vi "apresentacao.vi"() -> ()   [LabVIEW 2016]
uses:
  <vilib>/NXT/Subs/LVHSConnector.ctl
  <vilib>/NXT/LegoClasses/BrickReference/BrickReference.lvclass
  <vilib>/NXT/Block Support/NXT_InputPort.ctl
  <vilib>/NXT/Block Support/NXT_ButtonSelector.ctl
  <vilib>/NXT/Block Support/NXT_OutputPort.ctl
  <vilib>/NXT/Dual Mode Library/Advanced/NXTFlag_Clear.vi
  <vilib>/NXT/Dual Mode Library/Advanced/NXTFlag_Get_String.vi
  <vilib>/NXT/Dual Mode Library/Display/drawText_Center.vi
  <vilib>/NXT/Dual Mode Library/Advanced/NXTFlag_Get.vi
  <vilib>/NXT/Dual Mode Library/Advanced/NXTFlag_Clear_String.vi
  <vilib>/NXT/NXTIO Xnodes/NXTIONodeSubVIs/NXTMotorSteeringOn.vi
  <vilib>/NXT/NXTIO Xnodes/NXTIONodeSubVIs/NXTStopMotors.vi
  <vilib>/NXT/Dual Mode Library/Sensors/Sound_dBA.vi
  <vilib>/NXT/Dual Mode Library/Advanced/NXTFlag_Assign_String.vi
  <vilib>/NXT/Dual Mode Library/Sensors/Light_Off.vi
  <vilib>/NXT/Dual Mode Library/Sensors/Sonar_cm.vi
  <vilib>/NXT/Dual Mode Library/Sensors/Touch_Pressed.vi
  <vilib>/NXT/Dual Mode Library/Advanced/NXTFlag_Assign.vi
  <vilib>/NXT/Dual Mode Library/Sensors/readNXTButton.vi
  <vilib>/NXT/NXTIO Xnodes/AddressXNode/NXTIOAddress.xnode
  <vilib>/NXT/NXTIO Xnodes/NXTIOXNode/NXTIO.xnode
panel:
  out "NXT/EV3 2":T1
  in  "NXT/EV3":T1
  # "Entrada"
  # "Saída"
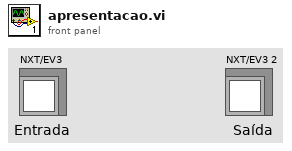
[diagram p1: front panel]
types:
  T1 = typedef "LVHSConnector.ctl" = refnum<class "BrickReference.lvclass">
  T2 = typedef "NXT_OutputPort.ctl" = u8
  T3 = typedef "NXT_ButtonSelector.ctl" = u16
  T4 = typedef "NXT_InputPort.ctl" = u32
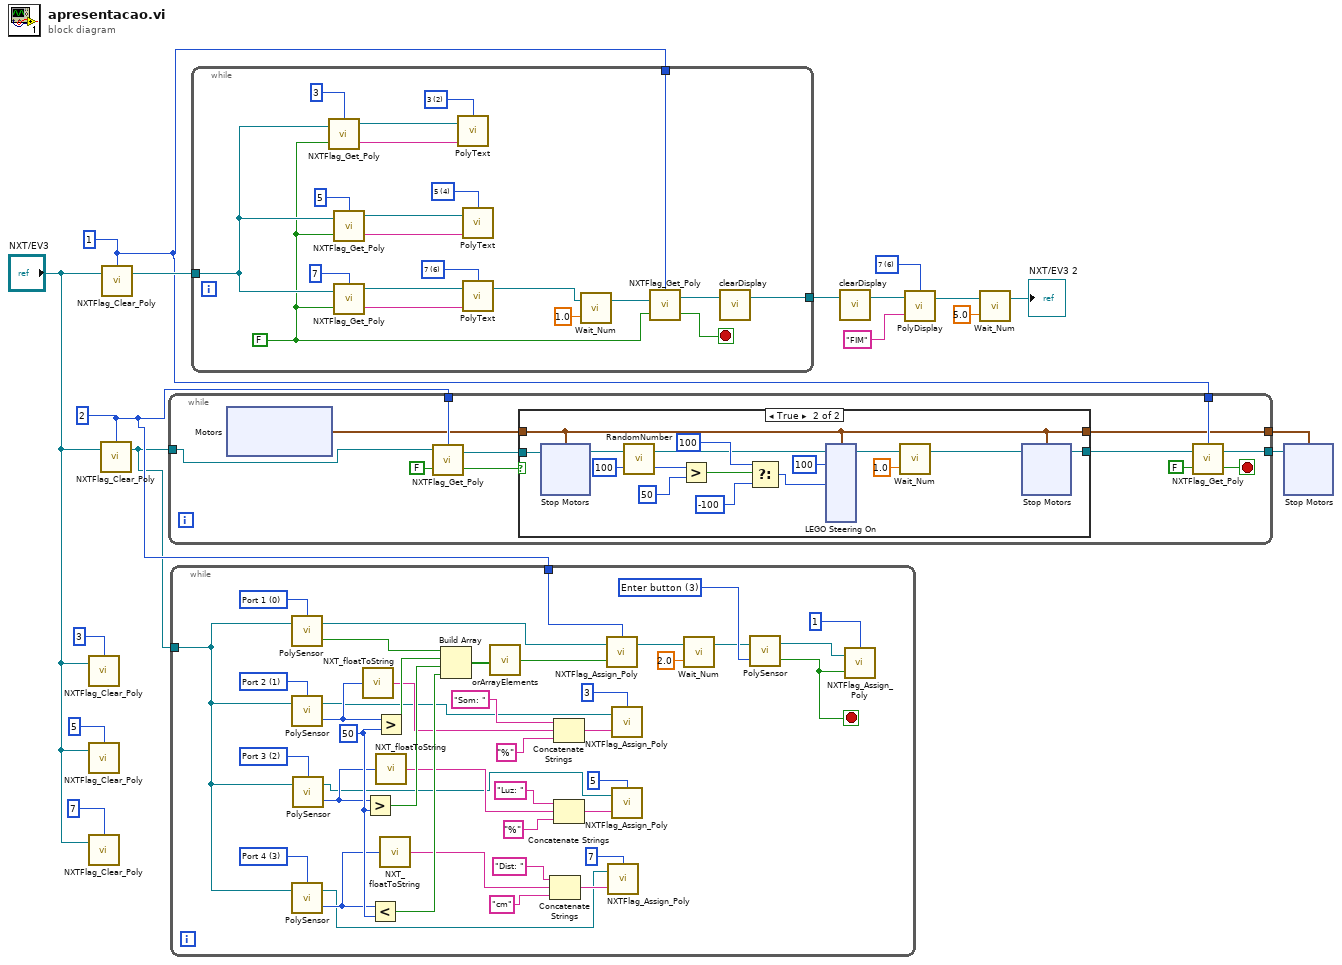
[diagram p0: block diagram]
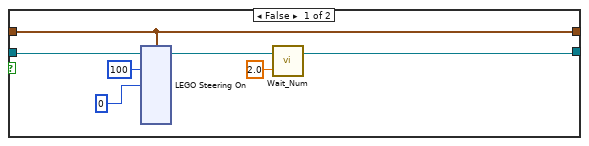
[diagram p2: hidden frame]
diagram:
  w5 = i16 6 items=["1", "2", "3", "4", "5", "6", "7", "8", "9", "10", "11", "12"] ("Line")
  w13 = 2 ("NXT/EV3 Flag Number")
  w12 = 1 ("NXT/EV3 Flag Number")
  n1 = call-poly <vilib>:"NXTFlag_Clear_Poly.vi"("NXT/EV3"="NXT/EV3", "NXT/EV3 Flag Number"=3) -> ()  [unwired: 2 in, 1 out]
  n2 = call-poly <vilib>:"NXTFlag_Clear_Poly.vi"("NXT/EV3"="NXT/EV3", "NXT/EV3 Flag Number"=5) -> ()  [unwired: 2 in, 1 out]
  n3 = call-poly <vilib>:"NXTFlag_Clear_Poly.vi"("NXT/EV3"="NXT/EV3", "NXT/EV3 Flag Number"=7) -> ()  [unwired: 2 in, 1 out]
  n4 = call-poly <vilib>:"NXTFlag_Clear_Poly.vi"("NXT/EV3"="NXT/EV3", "NXT/EV3 Flag Number"=w13) -> ("NXT/EV3"=w11:T1)  [unwired: 2 in]
  n5 = call-poly <vilib>:"NXTFlag_Clear_Poly.vi"("NXT/EV3"="NXT/EV3", "NXT/EV3 Flag Number"=w12) -> ("NXT/EV3"=w17:T1)  [unwired: 2 in]
  n6 = while {
    tunnel: w12 -> [w28]
    tunnel: w11 -> [w20]
    tunnel: w13 -> [w27]
    tunnel: [w22] -> w14
    tunnel: [w19] -> w6
    stop <- w29 stop-if-true
    n7 = xnode "Motors"() -> ("Motor"=w23:cluster{"Port":T2, "Port":T2})
    n8 = call-poly <vilib>:"NXTFlag_Get_Poly.vi"("Clear if Found"=FALSE, "NXT/EV3"=w20, "NXT/EV3 Flag Number"=w27) -> ("status"=w25:bool, "NXT/EV3"=w24:T1)
    n9 = case shown="True" w25 {
      tunnel: w24 -> [w35 w60]
      tunnel: w23 -> [w33 w49]
      tunnel: [w30 w59] -> w18
      tunnel: [w33 w49] -> w19
      frame False {
        n10 = xnode "LEGO Steering On"("Steering 1"=0, "Power 1"=100, "Motors"=w33, "NXT/EV3"=w35) -> ("NXT/EV3"=w31:T1)
        n11 = call <vilib>:"Wait_Num.vi"("Time (1 sec)"=sgl 2.0, "NXT/EV3"=w31) -> ("NXT/EV3"=w30:T1)  [unwired: 2 in]
      }
      frame True {
        n12 = xnode "Stop Motors"("Motors"=w49, "NXT/EV3"=w60) -> ("NXT/EV3"=w57:T1)
        n13 = call <vilib>:"RandomNumber.vi"("Max Value"=u16 100, "NXT"=w57) -> ("Random Number"=w55:u16, "NXT"=w48:T1)  [unwired: 1 in]
        n14 = Greater?(x=w55, y=u16 50) -> (0:w52:bool)
        n15 = Select(t=100 ("Steering 1"), s=w52, f=-100) -> (s? t:f=w53:i32)
        n16 = xnode "LEGO Steering On"("Steering 1"=w53, "Power 1"=100, "Motors"=w49, "NXT/EV3"=w48) -> ("NXT/EV3"=w46:T1)
        n17 = call <vilib>:"Wait_Num.vi"("Time (1 sec)"=sgl 1.0, "NXT/EV3"=w46) -> ("NXT/EV3"=w45:T1)  [unwired: 2 in]
        n18 = xnode "Stop Motors"("Motors"=w49, "NXT/EV3"=w45) -> ("NXT/EV3"=w59:T1)
      }
    }
    n19 = call-poly <vilib>:"NXTFlag_Get_Poly.vi"("Clear if Found"=FALSE, "NXT/EV3"=w18, "NXT/EV3 Flag Number"=w28) -> ("status"=w29:bool, "NXT/EV3"=w22:T1)
  }
  n20 = while {
    tunnel: w11 -> [w117]
    tunnel: w13 -> [w102]
    stop <- w105 stop-if-true
    w107 = T3 3 items=["Enter button"=3, "Left button"=2, "Right button"=1, "Up Button"=4, "Down Button"=5] ("Button (Enter button)")
    w112 = i16 50 ("y")
    w118 = T4 2 items=["Port 1", "Port 2", "Port 3", "Port 4"] ("Port (Port 3)")
    w119 = T4 1 items=["Port 1", "Port 2", "Port 3", "Port 4"] ("Port (Port 2)")
    w120 = T4 3 items=["Port 1", "Port 2", "Port 3", "Port 4"] ("Port (Port 4)")
    w121 = T4 0 items=["Port 1", "Port 2", "Port 3", "Port 4"] ("Port (Port 1)")
    n21 = call-poly <vilib>:"PolySensor.vi"("NXT/EV3"=w117, "Port (Port 1)"=w121) -> ("Yes / No"=w116:bool, "NXT/EV3"=w103:T1)  [unwired: 1 in]
    n22 = call-poly <vilib>:"PolySensor.vi"("NXT/EV3"=w117, "Port (Port 2)"=w119) -> ("sound (dBA)"=w111:i16, "NXT/EV3"=w83:T1)  [unwired: 1 in]
    n23 = call-poly <vilib>:"PolySensor.vi"("NXT/EV3"=w117, "Port (Port 4)"=w120) -> ("Distance (cm)"=w101:i16, "NXT/EV3"=w85:T1)  [unwired: 1 in]
    n24 = call-poly <vilib>:"PolySensor.vi"("NXT/EV3"=w117, "Port (Port 3)"=w118) -> ("Scaled Value"=w110:i16, "NXT/EV3"=w84:T1)  [unwired: 1 in]
    n25 = call <vilib>:"NXT_floatToString.vi"("number"=w111) -> ("string"=w87:string)
    n26 = Greater?(x=w110, y=w112) -> (0:w114:bool)
    n27 = Less?(x=w101, y=w112) -> (x < y?=w113:bool)
    n28 = Greater?(x=w111, y=w112) -> (0:w115:bool)
    n29 = call <vilib>:"NXT_floatToString.vi"("number"=w110) -> ("string"=w91:string)
    n30 = call <vilib>:"NXT_floatToString.vi"("number"=w101) -> ("string"=w93:string)
    n31 = Build Array(w116, w115, w114, w113) -> (w108:bool[])
    n32 = call <vilib>:"orArrayElements.vi"("Boolean Array"=w108) -> ("Logical OR"=w104:bool)
    n33 = Concatenate Strings("Dist: ", w93, "cm") -> (w98:string)
    n34 = Concatenate Strings("Som: ", w87, "%" ("string")) -> (w109:string)
    n35 = Concatenate Strings("Luz: ", w91, "%" ("string")) -> (w99:string)
    n36 = call-poly <vilib>:"NXTFlag_Assign_Poly.vi"("Flag State"=w104, "NXT/EV3"=w103, "NXT/EV3 Flag Number"=w102) -> ("NXT/EV3"=w81:T1)  [unwired: 1 in]
    n37 = call-poly <vilib>:"NXTFlag_Assign_Poly.vi"("Flag Value"=w98, "NXT/EV3"=w85, "NXT/EV3 Flag Number"=i8 7) -> ()  [unwired: 1 in, 1 out]
    n38 = call-poly <vilib>:"NXTFlag_Assign_Poly.vi"("Flag Value"=w109, "NXT/EV3"=w83, "NXT/EV3 Flag Number"=i8 3) -> ()  [unwired: 1 in, 1 out]
    n39 = call-poly <vilib>:"NXTFlag_Assign_Poly.vi"("Flag Value"=w99, "NXT/EV3"=w84, "NXT/EV3 Flag Number"=i8 5) -> ()  [unwired: 1 in, 1 out]
    n40 = call <vilib>:"Wait_Num.vi"("Time (1 sec)"=sgl 2.0, "NXT/EV3"=w81) -> ("NXT/EV3"=w80:T1)  [unwired: 2 in]
    n41 = call-poly <vilib>:"PolySensor.vi"("Button (Enter button)"=w107, "NXT/EV3"=w80) -> ("Yes/No"=w105:bool, "NXT/EV3"=w100:T1)  [unwired: 1 in]
    n42 = call-poly <vilib>:"NXTFlag_Assign_Poly.vi"("Flag State"=w105, "NXT/EV3"=w100, "NXT/EV3 Flag Number"=i8 1) -> ()  [unwired: 1 in, 1 out]
  }
  n43 = while {
    tunnel: w12 -> [w139]
    tunnel: w17 -> [w138]
    tunnel: [w123] -> w16
    stop <- w141 stop-if-true
    w131 = i16 6 items=["1", "2", "3", "4", "5", "6", "7", "8", "9", "10", "11", "12"] ("Line")
    w132 = i16 4 items=["1", "2", "3", "4", "5", "6", "7", "8", "9", "10", "11", "12"] ("Line")
    w137 = i16 2 items=["1", "2", "3", "4", "5", "6", "7", "8", "9", "10", "11", "12"] ("Line")
    w128 = FALSE ("Clear if Found")
    n44 = call-poly <vilib>:"NXTFlag_Get_Poly.vi"("Clear if Found"=w128, "NXT/EV3"=w138, "NXT/EV3 Flag Number"=3) -> ("Flag Value"=w136:string, "NXT/EV3"=w135:T1)
    n45 = call-poly <vilib>:"NXTFlag_Get_Poly.vi"("Clear if Found"=w128, "NXT/EV3"=w138, "NXT/EV3 Flag Number"=5) -> ("Flag Value"=w133:string, "NXT/EV3"=w134:T1)
    n46 = call-poly <vilib>:"NXTFlag_Get_Poly.vi"("Clear if Found"=w128, "NXT/EV3"=w138, "NXT/EV3 Flag Number"=7) -> ("Flag Value"=w130:string, "NXT/EV3"=w129:T1)
    n47 = call-poly <vilib>:"PolyText.vi"("Text"=w136, "NXT/EV3"=w135, "Line"=w137) -> ()  [unwired: 1 in, 1 out]
    n48 = call-poly <vilib>:"PolyText.vi"("Text"=w133, "NXT/EV3"=w134, "Line"=w132) -> ()  [unwired: 1 in, 1 out]
    n49 = call-poly <vilib>:"PolyText.vi"("Text"=w130, "NXT/EV3"=w129, "Line"=w131) -> ("NXT/EV3"=w127:T1)  [unwired: 1 in]
    n50 = call <vilib>:"Wait_Num.vi"("Time (1 sec)"=sgl 1.0, "NXT/EV3"=w127) -> ("NXT/EV3"=w140:T1)  [unwired: 2 in]
    n51 = call-poly <vilib>:"NXTFlag_Get_Poly.vi"("Clear if Found"=w128, "NXT/EV3"=w140, "NXT/EV3 Flag Number"=w139) -> ("status"=w141:bool, "NXT/EV3"=w122:T1)
    n52 = call <vilib>:"clearDisplay.vi"("NXT/EV3"=w122) -> ("NXT/EV3"=w123:T1)  [unwired: 3 in]
  }
  n53 = call <vilib>:"clearDisplay.vi"("NXT/EV3"=w16) -> ("NXT/EV3"=w15:T1)  [unwired: 3 in]
  n54 = call-poly <vilib>:"PolyDisplay.vi"("Text"="FIM", "NXT/EV3"=w15, "Line"=w5) -> ("NXT/EV3"=w2:T1)  [unwired: 1 in]
  n55 = call <vilib>:"Wait_Num.vi"("Time (1 sec)"=sgl 5.0, "NXT/EV3"=w2) -> ("NXT/EV3"=→"NXT/EV3 2":T1)  [unwired: 2 in]
  n56 = xnode "Stop Motors"("Motors"=w6, "NXT/EV3"=w14) -> ()  [unwired: 1 out]
